vi "Fake - 1 Session Unregistered 3 Sessions Registered Last Session Bad.vi"(8 "error in":errorcluster) -> (0 "error out":errorcluster, 3 "session reservation out":refnum<class "Session Reservation.lvclass">)   [LabVIEW 2020, in "MeasurementServerTests.lvlib"]
uses:
  MeasurementServerTests.lvlib
  Runtime/MeasurementLink Session Management/Session Reservation/Session Reservation.lvclass
  TestUtilities/TestUtilities.Runtime/Session Reservation Test Utilities/Session Reservation Test Utilities.lvlib
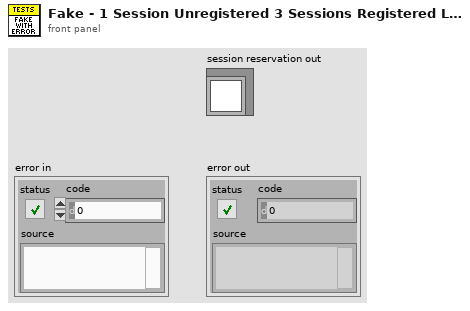
[diagram p1: front panel]
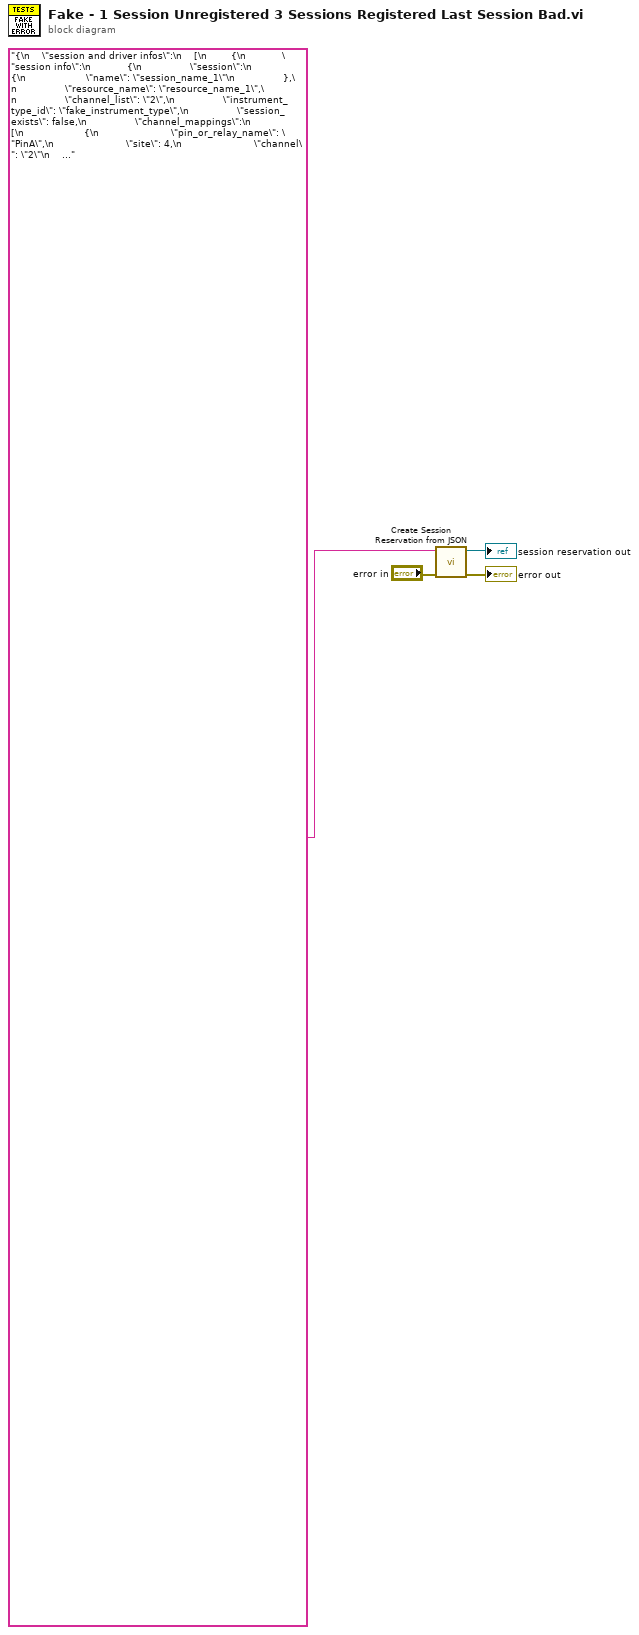
[diagram p0: block diagram]
diagram:
  n1 = call "Create Session Reservation from JSON.vi"("error in"="error in", "json"="{\n    \"session and driver infos\":\n    [\n        {\n            \"session info\":\n            {\n                \"session\":\n                {\n                    \"name\": \"session_name_1\"\n                },\n                \"resource_name\": \"resource_name_1\",\n                \"channel_list\": \"2\",\n                \"instrument_type_id\": \"fake_instrument_type\",\n                \"session_exists\": false,\n                \"channel_mappings\":\n                [\n                    {\n                        \"pin_or_relay_name\": \"PinA\",\n                        \"site\": 4,\n                        \"channel\": \"2\"\n                    }\n                ]\n            }\n        },\n        {\n            \"session info\":\n            {\n                \"session\":\n                {\n                    \"name\": \"session_name_2\"\n                },\n                \"resource_name\": \"resource_name_2\",\n                \"channel_list\": \"1\",\n                \"instrument_type_id\": \"fake_instrument_type\",\n                \"session_exists\": true,\n                \"channel_mappings\":\n                [\n                    {\n                        \"pin_or_relay_name\": \"PinB\",\n                        \"site\": 4,\n                        \"channel\": \"1\"\n                    }\n                ]\n            }\n        },\n        {\n            \"session info\":\n            {\n                \"session\":\n                {\n                    \"name\": \"session_name_3\"\n                },\n                \"resource_name\": \"resource_name_3\",\n                \"channel_list\": \"0\",\n                \"instrument_type_id\": \"fake_instrument_type\",\n                \"session_exists\": true,\n                \"channel_mappings\":\n                [\n                    {\n                        \"pin_or_relay_name\": \"PinC\",\n                        \"site\": 4,\n                        \"channel\": \"0\"\n                    }\n                ]\n            }\n        },\n        {\n            \"session info\":\n            {\n                \"session\":\n                {\n                    \"name\": \"session_name_4\"\n                },\n                \"resource_name\": \"trigger_error\",\n                \"channel_list\": \"0\",\n                \"instrument_type_id\": \"fake_instrument_type\",\n                \"session_exists\": true,\n                \"channel_mappings\":\n                [\n                    {\n                        \"pin_or_relay_name\": \"PinD\",\n                        \"site\": 4,\n                        \"channel\": \"3\"\n                    }\n                ]\n            }\n        }\n    ],\n    \"pin or relay names\":\n    [\n        \"PinA\",\n        \"PinB\",\n        \"PinC\",\n        \"PinD\"\n    ],\n    \"pin map context\":\n    {\n        \"pin_map_id\": \"pin_map_id_1\",\n        \"sites\":\n        [\n            4\n        ]\n    },\n    \"dvr valid\": true\n}") -> ("error out"=→"error out":errorcluster, "session reservation out"=→"session reservation out":refnum<class "Session Reservation.lvclass">)  [unwired: 7 in, 1 out]
